vi "p21.vi"() -> ()   [LabVIEW 2023]
panel:
  out "Waveform Chart":dbl(graph)
  in  "t0":dbl
  in  "tsim":dbl
  out "T":dbl
  out "ns":dbl
  in  "fs muestreo":dbl
  # "we are gonna make the formula ts/T + 1"
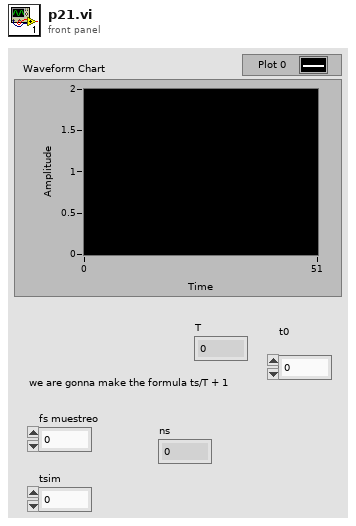
[diagram p1: front panel]
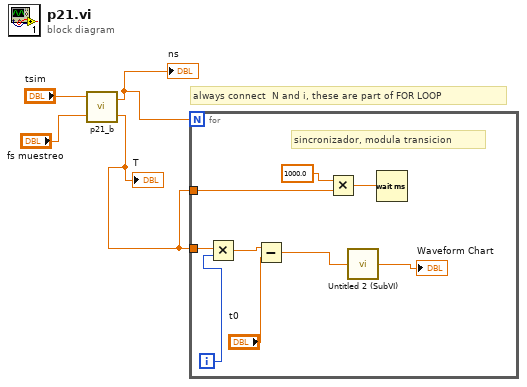
[diagram p0: block diagram]
diagram:
  # "always connect  N and i, these are part of FOR LOOP"
  n1 = call "p21_b.vi"("fs muestreo"="fs muestreo", "tsim"="tsim") -> ("T"=w2:dbl, "NS"=w1:dbl)
  "ns" <- w1
  "T" <- w2
  n2 = for {
    N: w1 -> [_]
    tunnel: w2 -> [w8]
    tunnel: w2 -> [w5]
    i -> [w7]
    # "sincronizador, modula transicion"
    n3 = Multiply(x=w8, y=w7) -> (x*y=w11:dbl)
    n4 = Subtract(x=w11, y="t0") -> (x-y=w9:dbl)
    n5 = Multiply(x=1000.0, y=w5) -> (x*y=w12:dbl)
    n6 = call "Untitled 2 (SubVI).vi"("input"=w9) -> ("output"=→"Waveform Chart":dbl)
    n7 = Wait (ms)(milliseconds to wait=w12) -> ()  [unwired: 1 out]
  }
